vi "ChangeHeadDir.vi"(8 "error in (no error)":errorcluster, 10 "UnitDirection":T1, 11 "2D_Representer in":refnum<class "2D_Representer.lvclass">) -> (0 "error out":errorcluster, 3 "2D_Representer out":refnum<class "2D_Representer.lvclass">)   [LabVIEW 2018, in "2D_Representer.lvclass"]
uses:
  2D_Representer.lvclass
  Typedefs/UnitDirection.ctl
  2D_Representer.lvclass/2D_Representer.ctl
  Snake/Snake.lvclass
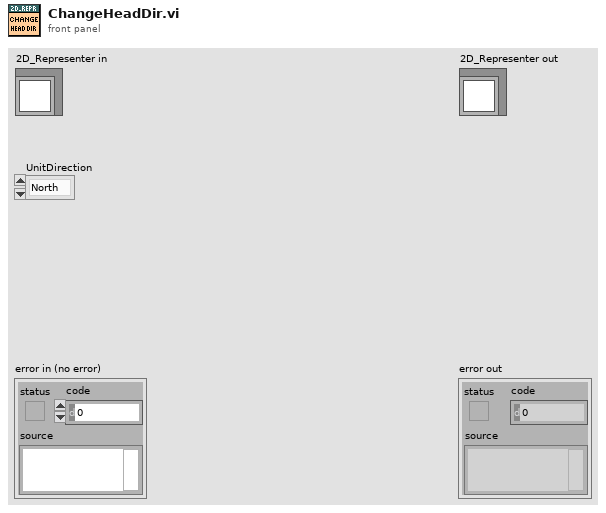
[diagram p1: front panel]
types:
  T1 = typedef "UnitDirection.ctl" = enum16{"North", "East", "South", "West"}
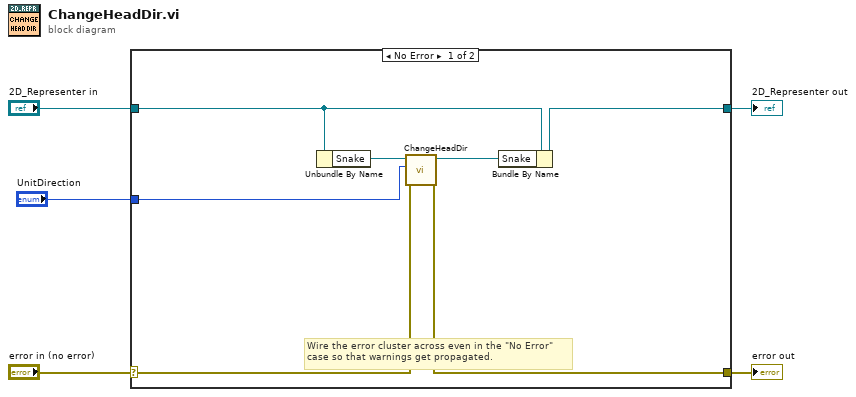
[diagram p0: block diagram]
diagram:
  n1 = case shown="No Error" "error in (no error)" {
    selector: "error in (no error)" -> [w7 w14]
    tunnel: [w6 w14] -> w4
    tunnel: [w11 w13] -> w2
    tunnel: "2D_Representer in" -> [w12 w13]
    tunnel: "UnitDirection" -> [w8 _]
    frame No Error {
      # "Wire the error cluster across even in the \"No Error\"\ncase so that warnings get propagated."
      n2 = Unbundle By Name(w12) -> ("Snake"=w10:refnum<class "Snake.lvclass">)
      n3 = call "ChangeHeadDir.vi"("error in (no error)"=w7, "UnitDirection"=w8, "Snake in"=w10) -> ("error out"=w6:errorcluster, "Snake out"=w9:refnum<class "Snake.lvclass">)  [unwired: 7 in]
      n4 = Bundle By Name(cluster=w12, "Snake"=w9) -> (w11:refnum<class "2D_Representer.lvclass">)
    }
    frame Error {
    }
  }
  "error out" <- w4
  "2D_Representer out" <- w2
